vi "connect.vi"() -> ()   [LabVIEW 2017]
uses:
  state_enum.ctl
  Global_BOC (SubVI).vi
  Unicorn Labview Library/Unicorn Library.lvlib
  <instrlib>/Siglent SDG X Series/Siglent SDG X Series.lvlib
  <instrlib>/PICOTEST M352XA/Public/Controls/Function.ctl
panel:
  in  "Tab Control":enum32{"Connect", "BOC-setup"}(tab)
  in  "Connect":bool
  out "Table Control":string[][](table)
  in  "voltmetr":refnum<visa-resource-name>
  in  "generator":refnum<visa-resource-name>
  in  "OK Button":bool
  out "Measurements":dbl[](array[numeric])
  in  "stop":bool
  out "error out":errorcluster
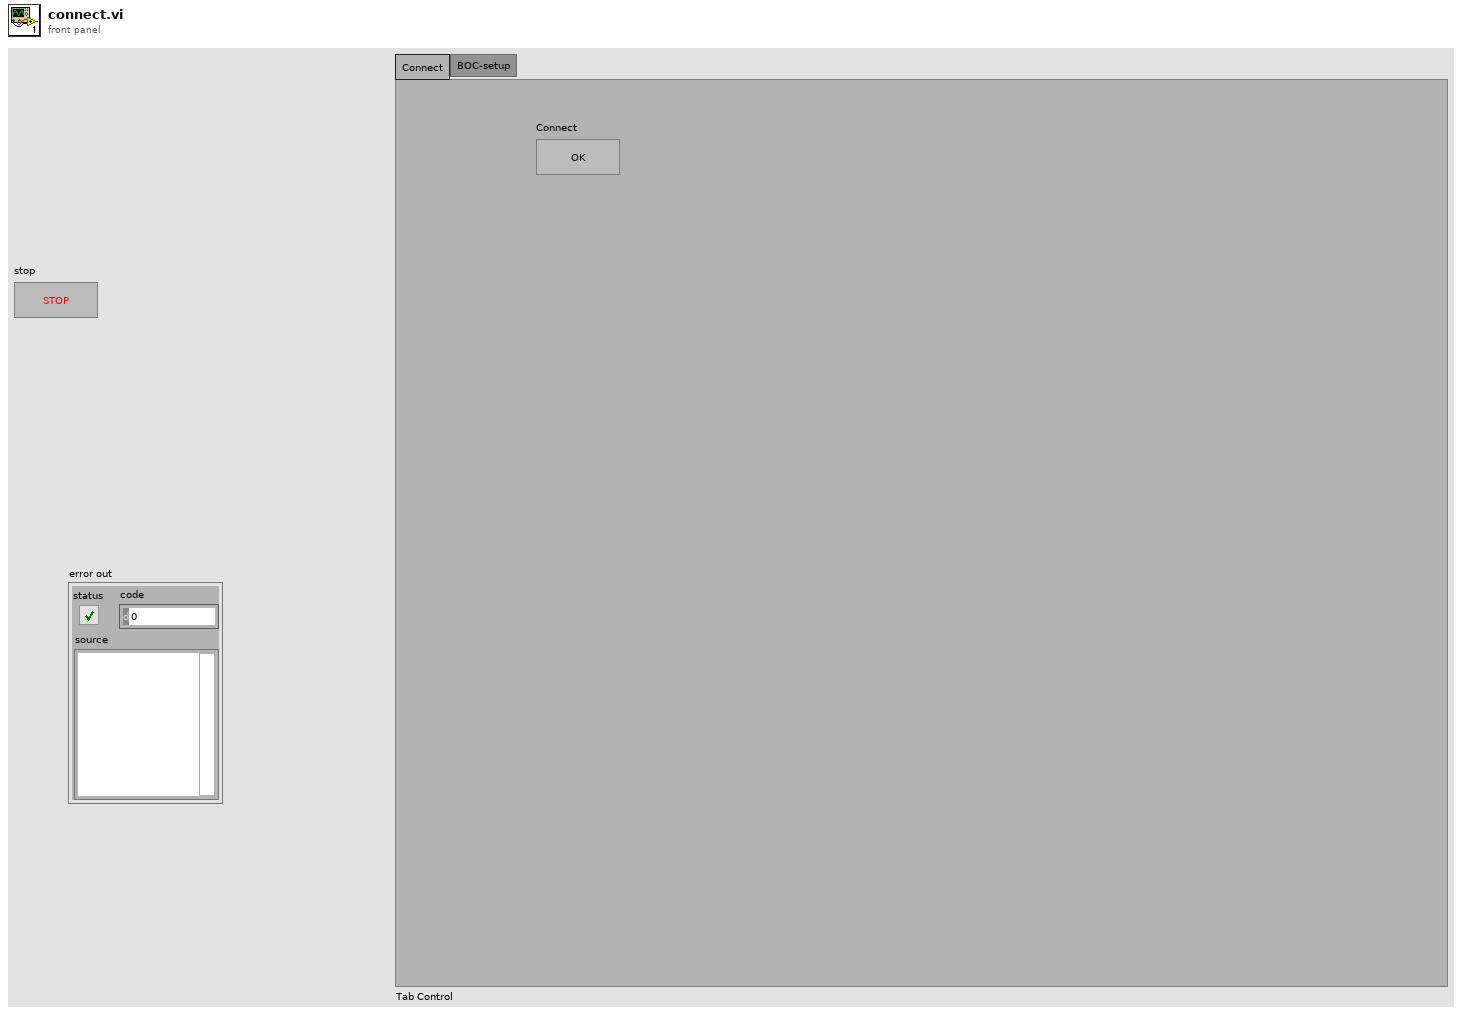
[diagram p1: front panel]
types:
  T1 = enum32{"Page Enabled", "Page Disabled", "Page Disabled & Grayed"}
  T2 = typedef "state_enum.ctl" = enum16{"Connect", "setup_devices", "setup_BOC", "measurments", "close"}
  T3 = typedef "Function.ctl" = enum16{"VOLTage:DC", "VOLTage:DC:RATio", "VOLTage:AC", "CURRent:DC", "CURRent:AC", "RESistance", "FRESistance", "FREQuency", "PERiod", "FREQuency:CURRent", "PERiod:CURRent", "CAPacitance", "CONTinuity", "DIODe", "TCOuple", "TEMPerature"}
  T4 = typedef "paramUnicorn.ctl" = cluster{"conParam":T5, "Param":T6}
  T5 = typedef "Unicorn Library.lvlib/connectionParam.ctl" = cluster{"ReadIntParam":bool, "ReadDescrParam":bool, "ReadFloatParam":bool, "debug":bool, "ReadJSON":bool, "IP_address":string, "N_attempts":i32, "type_con":enum16{"Serial", "TCP"}, "MB_address":i32, "VISA":refnum<visa-resource-name>, "connection ID":refnum<k5>, "nameDevices":string, "timeout":i32, "port":u16, "type_version":string, "baud_rate":u32, "VersionControl":bool, "TCP_conn":bool}
  T6 = typedef "Unicorn Library.lvlib/JSONParam.ctl" = cluster{"ParamInt":string[][], "ParamTelemetry":string[][], "ParamFloat":string[][], "TableCount":i32[][], "NeedParamPrepare":bool[], "NumParam":cluster{"NTelem":i32, "NInt":i32, "NFloat":i32}, "NTable":i32}
  T7 = typedef "Unicorn Library.lvlib/unicorn_Param.ctl" = cluster{"conParam":T8, "Param":T9}
  T8 = typedef "Unicorn Library.lvlib/unicorn_conn.ctl" = cluster{"ReadIntParam":bool, "ReadDescrParam":bool, "ReadFloatParam":bool, "debug":bool, "ReadJSON":bool, "IP_address":string, "N_attempts":i32, "type_con":enum16{"Serial", "TCP"}, "MB_address":i32, "VISA":refnum<visa-resource-name>, "connection ID":refnum<k5>, "nameDevices":string, "timeout":i32, "port":u16, "type_version":string, "baud_rate":u32, "VersionControl":bool, "TCP_conn":bool}
  T9 = typedef "Unicorn Library.lvlib/unicorn_JSON.ctl" = cluster{"NumParam":cluster{"NTelem":i32, "NInt":i32, "NFloat":i32, "NTable":i32}, "ParamInt":T10, "Telemetry":T11, "Table":T12, "ParamFloat":T13}
  T10 = typedef "Unicorn Library.lvlib/unicorn_ParamInt.ctl" = cluster{"ID":string, "Num":i32, "Name":string, "Type":string, "Enum":string, "Desc":string, "Unit":string, "Access":string, "FormatStr":string, "Min":i32, "Max":i32}[]
  T11 = typedef "Unicorn Library.lvlib/unicorn_Telemetry.ctl" = cluster{"ID":string, "Num":i32, "Name":string, "Desc":string, "Unit":string, "FormatStr":string, "Min":i32, "Max":i32}[]
  T12 = typedef "Unicorn Library.lvlib/unicorn_Table.ctl" = cluster{"Num":i32, "Access":string, "ColumnCount":i32, "NeedParamPrepare":bool, "Columns":cluster{"Column":i32, "Desc":string, "Name":string}[], "DataType":string, "FormatStr":string, "ID":string, "Name":string, "RowCount":i32, "Rows":cluster{"Desc":string, "ID":string, "Max":i32, "Min":i32, "Name":string, "Row":i32, "Unit":string}[], "Type":string}[]
  T13 = typedef "Unicorn Library.lvlib/unicorn_ParamFloat.ctl" = cluster{"ID":string, "Num":i32, "Name":string, "Type":string, "Enum":string, "Desc":string, "Unit":string, "Access":string, "FormatStr":string, "Min":i32, "Max":i32}[]
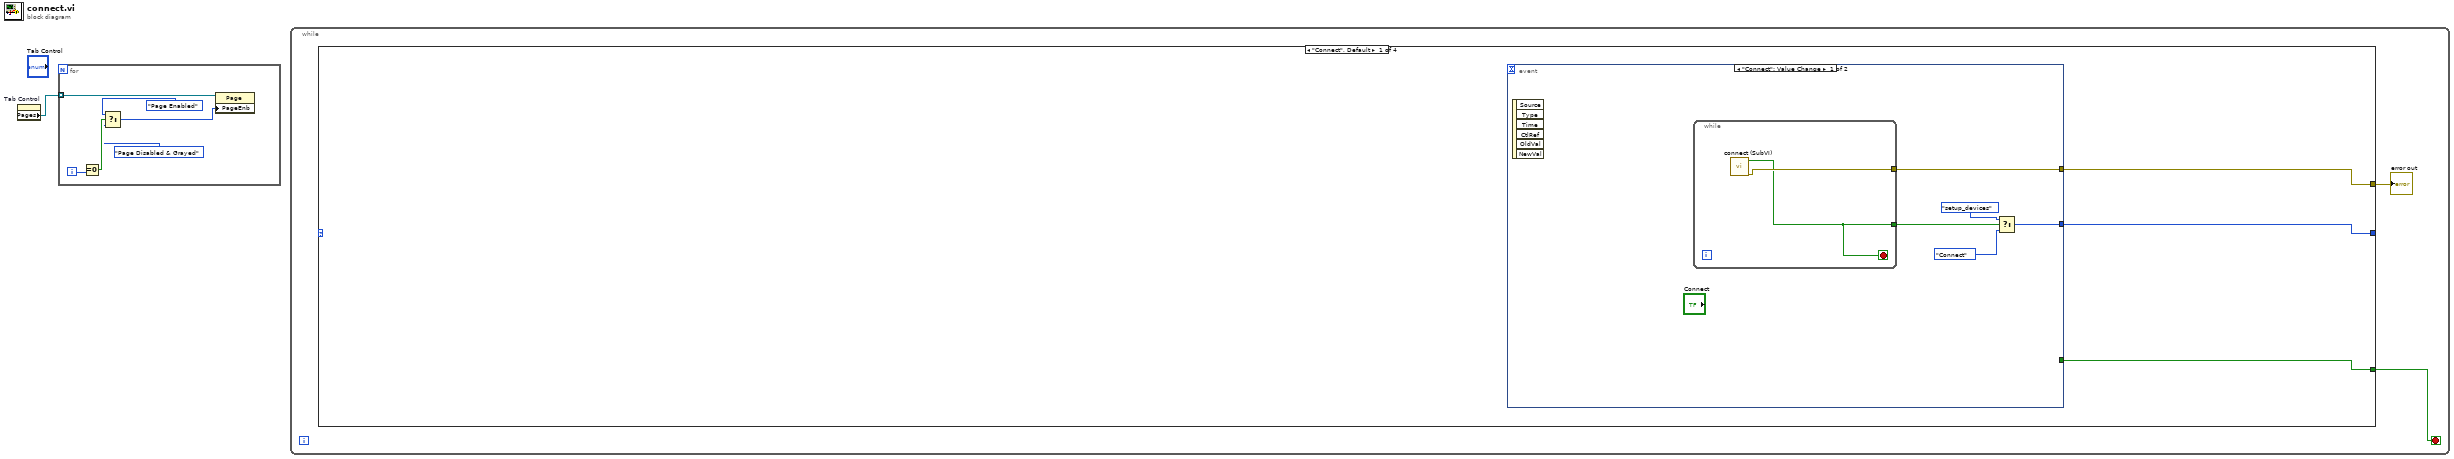
[diagram p0: block diagram]
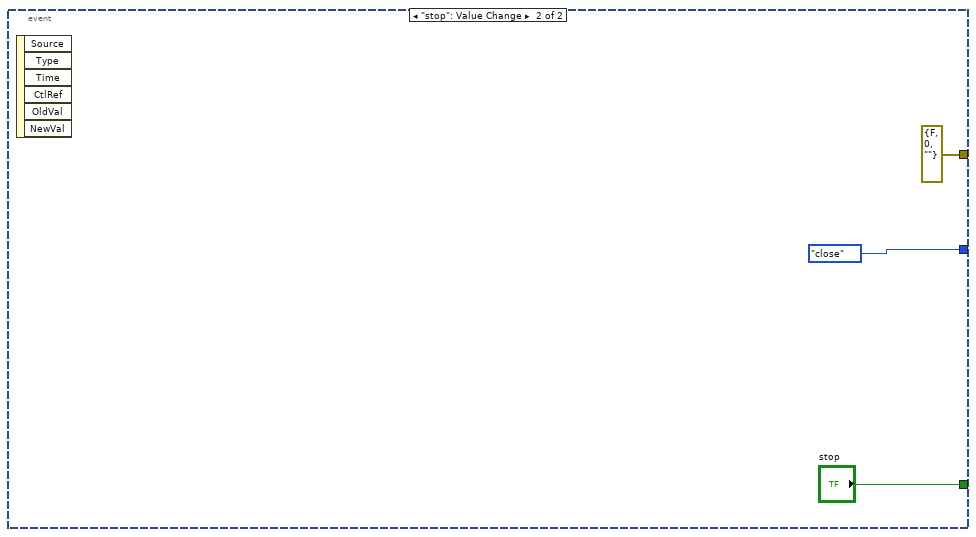
[diagram p2: hidden frame]
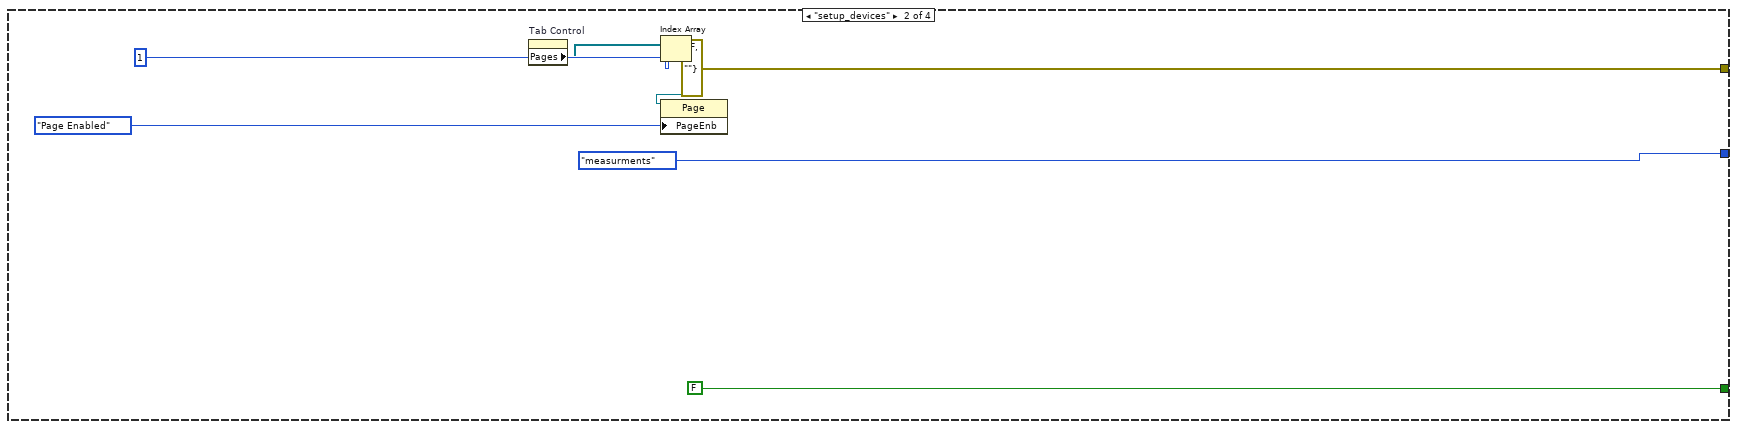
[diagram p3: hidden frame]
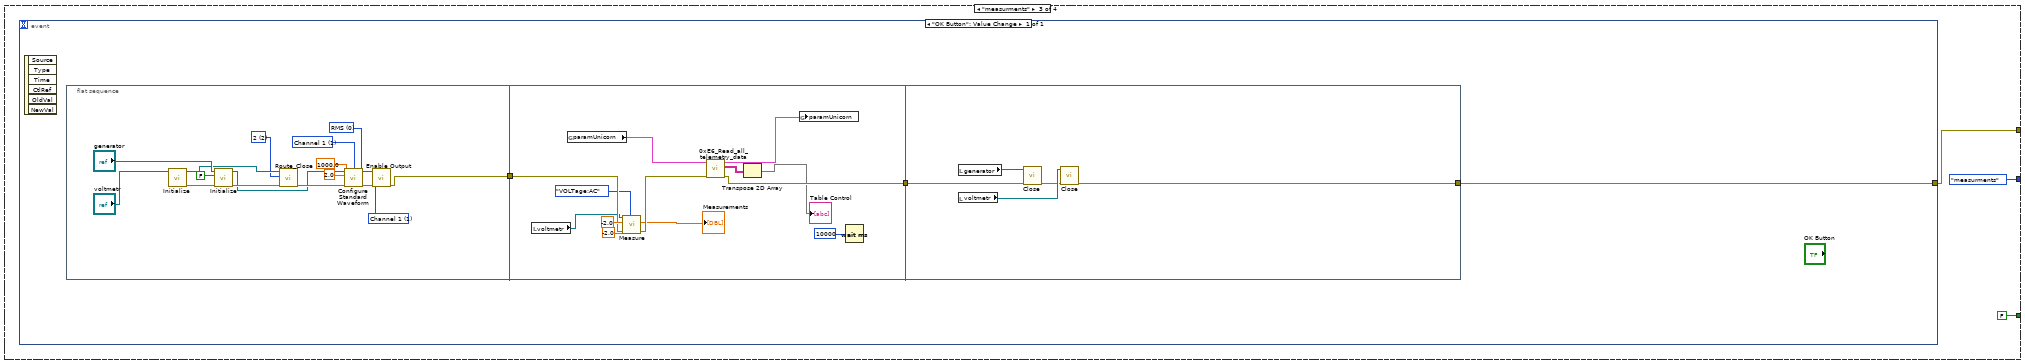
[diagram p4: hidden frame]
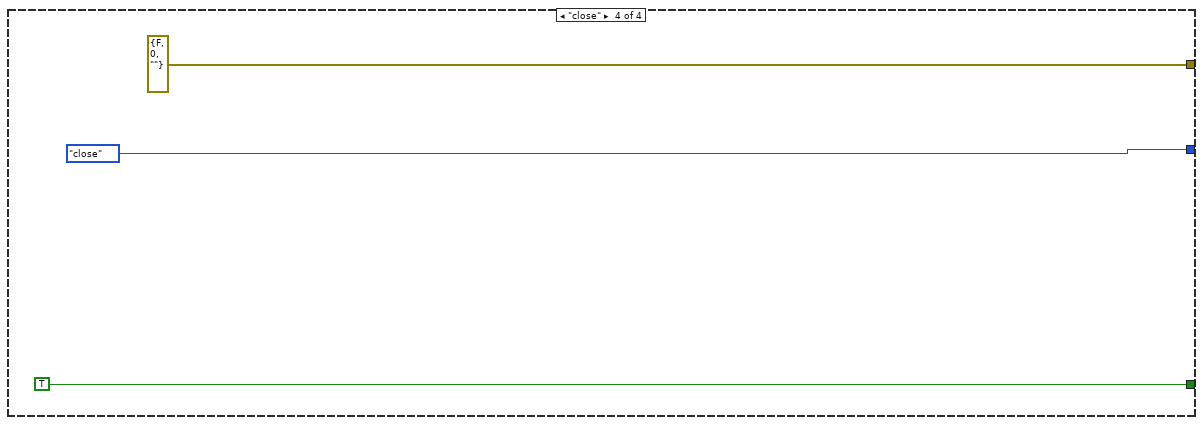
[diagram p5: hidden frame]
diagram:
  n1 = property on="Tab Control" class="TabCtl (strict)"() -> ("Pages"=w1:refnum<vi>[])  [unwired: 2 in, 2 out]
  n2 = for {
    tunnel: w1 -> [w7] mode=indexing
    i -> [w6]
    n3 = Equal To 0?(x=w6) -> (x = 0?=w5:bool)
    n4 = Select(t=T1."Page Enabled" ("Page Enabled State"), s=w5, f=T1."Page Disabled & Grayed" ("Page Enabled State")) -> (s? t:f=w3:T1)
    n5 = property class="Page"(reference=w7, "PageEnb"=w3) -> ()  [unwired: 1 in, 2 out]
  }
  n6 = while {
    stop <- w9 stop-if-true
    n7 = case shown="\"Connect\", Default" {
      selector: _ -> [_ _ _ _]
      tunnel: [w11 errorcluster {"status"=FALSE, "code"=0, "source"=""} ("error out") w31 errorcluster {"status"=FALSE, "code"=0, "source"=""} ("error out")] -> w10
      tunnel: [w13 FALSE ("stop") FALSE ("stop") TRUE ("stop")] -> w9
      tunnel: [w12 state_enum."measurments" state_enum."measurments" state_enum."close"] -> w8
      frame "Connect", Default {
        n8 = event shown="[0] \"Connect\": Value Change" {
          selector: _ -> [_ _]
          dyn-events: _ -> [_ _]
          timeout: _ -> [_ _]
          tunnel: [w18 errorcluster {"status"=FALSE, "code"=0, "source"=""} ("error out")] -> w11
          tunnel: [_ "stop"] -> w13
          tunnel: [w17 state_enum."close"] -> w12
          event "Connect": Value Change {
            n9 = event-data() -> ()  [unwired: 1 in, 6 out]
            n10 = while {
              tunnel: [w20] -> w18
              tunnel: [w19] -> w14
              stop <- w19 stop-if-true
              n11 = call "connect (SubVI).vi"() -> ("error out"=w20:errorcluster, "x != 0?"=w19:bool)  [unwired: 10 in]
            }
            n12 = Select(t=state_enum."setup_devices", s=w14, f=state_enum."Connect") -> (s? t:f=w17:T2)
          }
          event "stop": Value Change {
            n13 = event-data() -> ()  [unwired: 1 in, 6 out]
          }
        }
      }
      frame "setup_devices" {
        n14 = property on="Tab Control" class="TabCtl (strict)"() -> ("Pages"=w24:refnum<vi>[])  [unwired: 2 in, 2 out]
        n15 = Index Array(array=w24, index=1) -> (element=w25:refnum<vi>)
        n16 = property class="Page"(reference=w25, "PageEnb"=T1."Page Enabled" ("Page Enabled State")) -> ()  [unwired: 1 in, 2 out]
      }
      frame "measurments" {
        n17 = event shown="[0] \"OK Button\": Value Change" {
          selector: _ -> [_]
          dyn-events: _ -> [_]
          timeout: _ -> [_]
          tunnel: [w36] -> w31
          event "OK Button": Value Change {
            n18 = event-data() -> ()  [unwired: 1 in, 6 out]
            n19 = flat-sequence {
              tunnel: [w38] -> w34
              tunnel: [w63] -> w35
              tunnel: w34 -> [w59]
              tunnel: [w67] -> w36
              tunnel: w35 -> [w69]
              frame #0 {
                w39 = 1 items=["Channel 1"=1, "Channel 2"=2] ("Channel (1:Channel 1)")
                w40 = 1 items=["Channel 1"=1, "Channel 2"=2] ("Channel (1:Channel 1)")
                w44 = u16 0 items=["RMS", "pp", "dBm"] ("v-type")
                w48 = u8 2 items=["1"=1, "2"=2, "3"=3, "4"=4, "5"=5, "6"=6, "7"=7, "8"=8, "9"=9, "10"=10, "11"=11, "12"=12, "13"=13, "14"=14, "15"=15, "16"=16, "17"=17, "18"=18, "19"=19, "20"=20] ("channel")
                n20 = call <instrlib>:"Initialize.vi"("VISA resource name"="voltmetr") -> ("error out"=w53:errorcluster, "VISA resource name out"=w50:refnum<visa-resource-name>)  [unwired: 8 in, 1 out]
                n21 = call <instrlib>:"Initialize.vi"("error in (no error)"=w53, "ID Query (True)"=FALSE, "VISA resource name"="generator") -> ("error out"=w49:errorcluster, "VISA resource name out"=w46:refnum<visa-resource-name>)  [unwired: 7 in]
                n22 = call <instrlib>:"Route_Close.vi"("error in (no error)"=w49, "channel"=w48, "VISA resource name"=w50) -> ("error out"=w47:errorcluster)  [unwired: 6 in, 2 out]
                n23 = call <instrlib>:"Configure Standard Waveform.vi"("VISA resource name"=w46, "Channel (1:Channel 1)"=w39, "Amplitude (1.0 Vpp)"=2.0, "Frequency (1000 Hz)"=1000.0, "v-type"=w44, "error in (no error)"=w47) -> ("VISA resource name out"=w41:refnum<visa-resource-name>, "error out"=w42:errorcluster)  [unwired: 8 in]
                n24 = call <instrlib>:"Enable Output.vi"("error in (no error)"=w42, "Channel (1:Channel 1)"=w40, "VISA resource name"=w41) -> ("error out"=w38:errorcluster)  [unwired: 7 in, 1 out]
              }
              frame #1 {
                n25 = local read "voltmetr"() -> (w55:refnum<visa-resource-name>)
                n26 = global read "Global_BOC (SubVI).vi" "paramUnicorn"() -> (w65:T4)
                n27 = call <instrlib>:"Measure.vi"("Function"=Function."VOLTage:AC", "error in (no error)"=w59, "Resolution"=-2.0, "Range"=-2.0, "VISA resource name"=w55) -> ("error out"=w58:errorcluster, "Measurements"=→"Measurements":dbl[])  [unwired: 4 in, 1 out]
                n28 = call "0xE6_Read_all_telemetry_data.vi"("error in"=w58, "paramUnicorn"=w65) -> ("error out"=w63:errorcluster, "TblTelemetry"=w64:string[][], "paramUnicorn 2"=w66:T7)  [unwired: 4 in, 2 out]
                n29 = Transpose 2D Array(2D array=w64) -> (transposed array=→"Table Control":string[][])
                n30 = global write "Global_BOC (SubVI).vi" "paramUnicorn"(w66) -> ()
                n31 = Wait (ms)(milliseconds to wait=u32 10000) -> ()  [unwired: 1 out]
              }
              frame #2 {
                n32 = local read "generator"() -> (w71:refnum<visa-resource-name>)
                n33 = local read "voltmetr"() -> (w70:refnum<visa-resource-name>)
                n34 = call <instrlib>:"Close.vi"("error in (no error)"=w69, "VISA resource name"=w71) -> ("error out"=w68:errorcluster)  [unwired: 9 in]
                n35 = call <instrlib>:"Close.vi"("error in (no error)"=w68, "VISA resource name"=w70) -> ("error out"=w67:errorcluster)  [unwired: 9 in]
              }
            }
          }
        }
      }
      frame "close" {
      }
    }
    "error out" <- w10
  }
